vi "Measure.vi"(8 "error in (no error)":errorcluster, 11 "Prototype Measurement in":refnum<class "Prototype Measurement.lvclass">) -> (0 "error out":errorcluster, 3 "Prototype Measurement out":refnum<class "Prototype Measurement.lvclass">)   [LabVIEW 2013]
uses:
  <userlib>/Common Components/Results/Results.lvclass
  Result/Prototype Result.lvclass
  <userlib>/Common Components/Measurement Actor/Measurement.lvclass
  Measurement/Prototype Measurement.lvclass
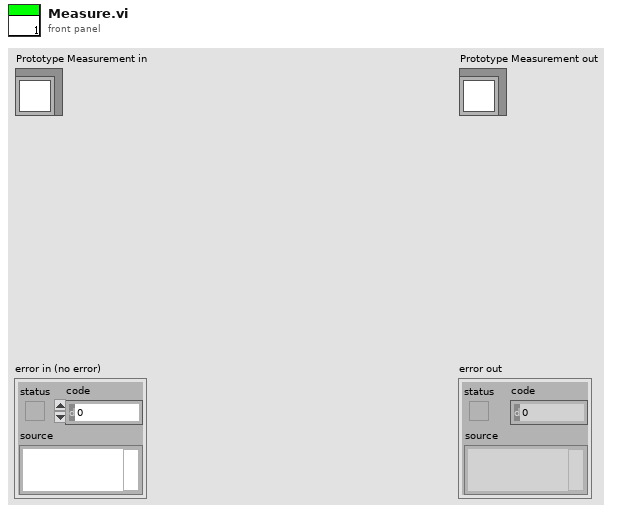
[diagram p1: front panel]
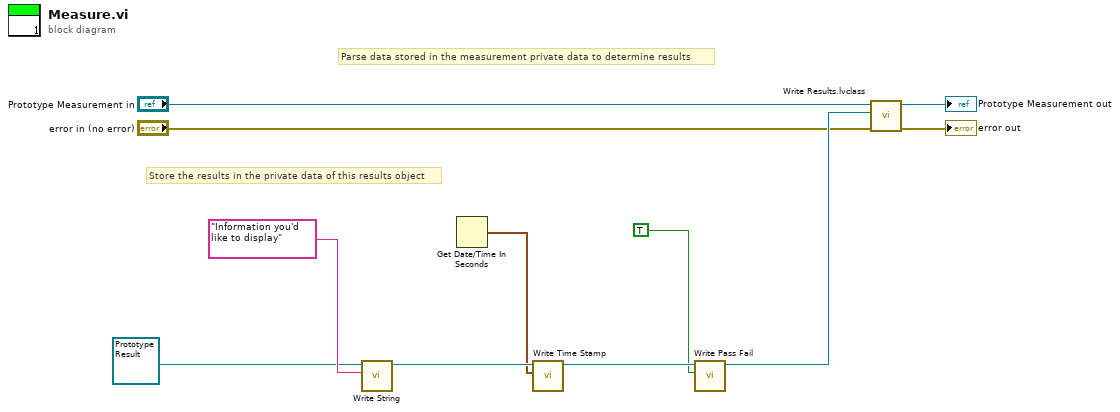
[diagram p0: block diagram]
diagram:
  # "Store the results in the private data of this results object"
  # "Parse data stored in the measurement private data to determine results"
  n1 = call <userlib>:"Write String.vi"("String"="Information you'd like to display", "Results in"=refnum<class "Prototype Result.lvclass"> refnum ("Prototype Result.lvclass")) -> ("Results out"=w11:refnum<class "Prototype Result.lvclass">)  [unwired: 8 in, 1 out]
  n2 = Get Date/Time In Seconds() -> (seconds since 1Jan1904=w8:timestamp)
  n3 = call <userlib>:"Write Time Stamp.vi"("Time Stamp"=w8, "Results in"=w11) -> ("Results out"=w10:refnum<class "Prototype Result.lvclass">)  [unwired: 8 in, 1 out]
  n4 = call <userlib>:"Write Pass Fail.vi"("Pass Fail"=TRUE, "Results in"=w10) -> ("Results out"=w3:refnum<class "Prototype Result.lvclass">)  [unwired: 8 in, 1 out]
  n5 = call <userlib>:"Write Results.lvclass.vi"("error in (no error)"="error in (no error)", "Result Actor.lvlib:Results.lvclass"=w3, "Measurement in"="Prototype Measurement in") -> ("error out"=→"error out":errorcluster, "Measurement out"=→"Prototype Measurement out":refnum<class "Prototype Measurement.lvclass">)  [unwired: 7 in]
